vi "Cull and Group Peg.vi"(9 "Score Cutoff":dbl=3.0, 10 "Sorted Data":dbl[][](array[numeric])) -> (0 "Rect":T1, 1 "Line":T1, 2 "Score":dbl, 3 "Center":cluster{"X":dbl, "Y":dbl})   [LabVIEW 2016]
doc: "Examine the particle measurements to find the most likely pair that make up the target. This mostly compares the edges of the bounding boxes. It then returns information about the overall target, notably the rectangle sourrounding the particles, the vertical line that bisects the target, and the center of the top particle."
panel:
  out "Grouping Scores":T2(array[cluster])
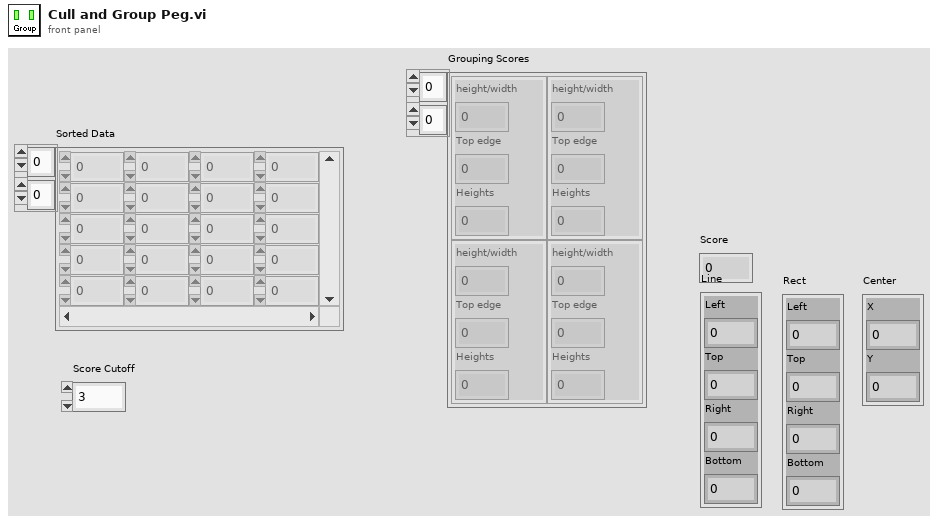
[diagram p1: front panel]
types:
  T1 = cluster{"Left":dbl, "Top":dbl, "Right":dbl, "Bottom":dbl}
  T2 = cluster{"height/width":dbl, "Top edge":dbl, "Heights":dbl}[][]
  T3 = cluster{"height/width":dbl, "Top edge":dbl, "Heights":dbl}
  T4 = cluster{"Left":dbl, "Numeric":dbl, "Right":dbl, "Numeric":dbl}
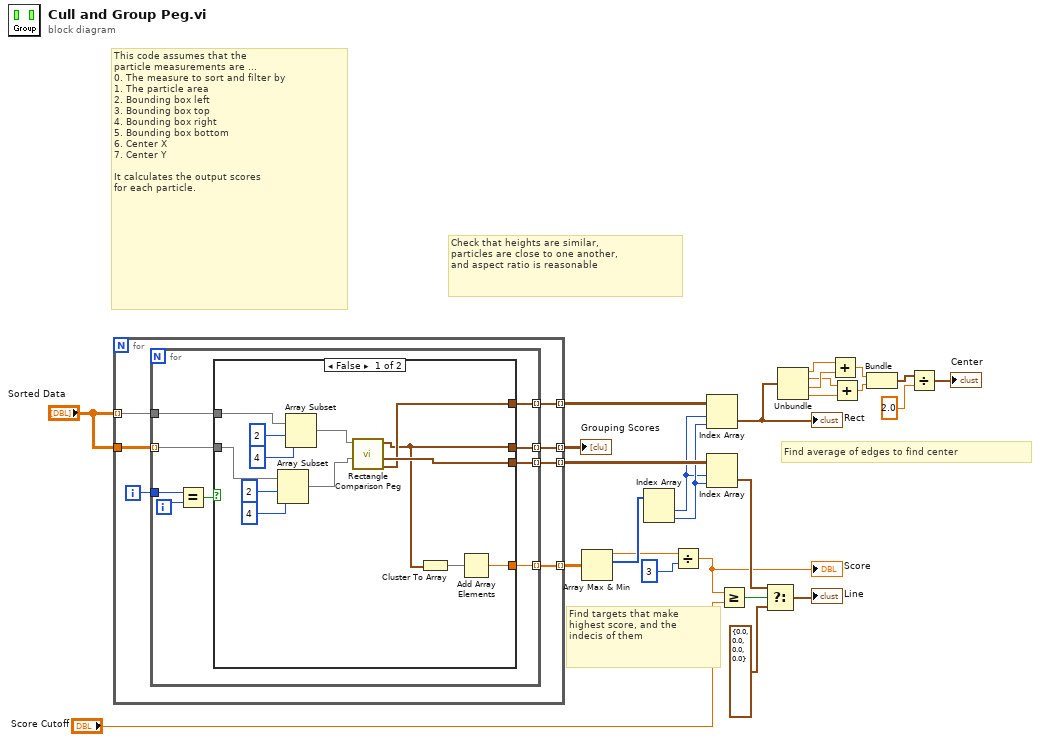
[diagram p0: block diagram]
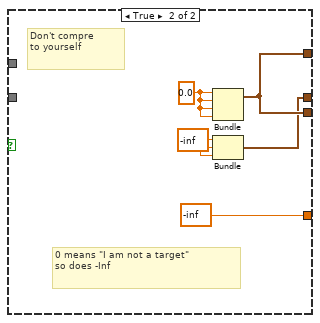
[diagram p2: hidden frame]
diagram:
  # "Find targets that make\nhighest score, and the\nindecis of them"
  # "Find average of edges to find center"
  # "Check that heights are similar,\nparticles are close to one another, \nand aspect ratio is reasonable"
  # "This code assumes that the\nparticle measurements are ...\n0. The measure to sort and filter by\n1. The particle area\n2. Bounding box left\n3. Bounding box top\n4. Bounding box right\n5. Bounding box bottom\n6. Center X\n7. Center Y\n\nIt calculates the output scores\nfor each particle."
  n1 = for {
    tunnel: "Sorted Data" -> [w33] mode=indexing
    tunnel: "Sorted Data" -> [w32]
    tunnel: [w30] -> w26 mode=indexing
    tunnel: [w29] -> w23 mode=indexing
    tunnel: [w28] -> w19 mode=indexing
    tunnel: [w27] -> w12 mode=indexing
    i -> [w31]
    n2 = for {
      tunnel: w33 -> [w42]
      tunnel: w32 -> [w40] mode=indexing
      tunnel: w31 -> [w39]
      tunnel: [w37] -> w30 mode=indexing
      tunnel: [w36] -> w29 mode=indexing
      tunnel: [w35] -> w28 mode=indexing
      tunnel: [w34] -> w27 mode=indexing
      i -> [w38]
      n3 = Equal?(x=w39, y=w38) -> (x = y?=w41:bool)
      n4 = case shown="False" w41 {
        tunnel: w42 -> [w53 _]
        tunnel: w40 -> [w50 _]
        tunnel: [w48 -inf] -> w37
        tunnel: [w45 w59] -> w36
        tunnel: [w44 w59] -> w35
        tunnel: [w43 w56] -> w34
        frame False {
          n5 = Array Subset(array=w50, index=2, length=4) -> (w47:dbl[])
          n6 = Array Subset(array=w53, index=2, length=4) -> (w46:dbl[])
          n7 = call "Rectangle Comparison Peg.vi"("Second"=w47, "First"=w46) -> ("Rect"=w44:T1, "Line"=w45:T1, "Scores"=w43:T3)  [unwired: 7 in]
          n8 = Cluster To Array(cluster=w43) -> (array=w49:dbl[])
          n9 = Add Array Elements(numeric array=w49) -> (sum=w48:dbl)
        }
        frame True {
          w57 = -inf
          w58 = 0.0
          # "0 means \"I am not a target\"\nso does -Inf"
          # "Don't compre\nto yourself"
          n10 = Bundle(w58, w58, w58, w58) -> (w59:cluster{dbl, dbl, dbl, dbl})  [unwired: 1 in]
          n11 = Bundle(w57, w57, w57) -> (w56:cluster{dbl, dbl, dbl})  [unwired: 1 in]
        }
      }
    }
  }
  "Grouping Scores" <- w12
  n12 = Array Max & Min(array=w26) -> (max value=w14:dbl, max index (indices)=w15:i32[])  [unwired: 2 out]
  n13 = Index Array(array=w15) -> (element #1=w16:i32, element #2=w18:i32)  [unwired: 2 in]
  n14 = Divide(x=w14, y=3 ("index")) -> (x/y=w13:dbl)
  "Score" <- w13
  n15 = Index Array(array=w19, index (row)=w16, index (col)=w18) -> (element=w11:T1)
  "Rect" <- w11
  n16 = Index Array(array=w23, index (row)=w16, index (col)=w18) -> (element=w22:T1)
  n17 = Greater Or Equal?(x=w13, y="Score Cutoff") -> (x >= y?=w25:bool)
  n18 = Select(t=w22, s=w25, f=cluster{dbl, "Numeric":dbl, dbl, "Numeric":dbl} {0.0, "Numeric"=0.0, 0.0, "Numeric"=0.0}) -> (s? t:f=→"Line":T4)
  n19 = Unbundle(w11) -> ("Left"=w10:dbl, "Top"=w2:dbl, "Right"=w9:dbl, "Bottom"=w7:dbl)
  n20 = Add(x=w10, y=w9) -> (x+y=w8:dbl)
  n21 = Add(x=w2, y=w7) -> (x+y=w6:dbl)
  n22 = Bundle(w8, w6) -> (w5:cluster{dbl, dbl})  [unwired: 1 in]
  n23 = Divide(x=w5, y=2.0) -> (x/y=→"Center":cluster{dbl, dbl})
